vi "M04 Smart Grid.vi"(11 "EV3 in":T1) -> (3 "EV3 out":T1)   [LabVIEW 2016]
uses:
  <vilib>/NXT/Subs/LVHSConnector.ctl
  <vilib>/NXT/LegoClasses/BrickReference/BrickReference.lvclass
  <vilib>/NXT/Block Support/NXT_OutputPort.ctl
  <vilib>/NXT/NXTIO Xnodes/NXTIONodeSubVIs/NXTMotorRunDistance.vi
  <vilib>/NXT/NXTIO Xnodes/AddressXNode/NXTIOAddress.xnode
  <vilib>/NXT/NXTIO Xnodes/NXTIOXNode/NXTIO.xnode
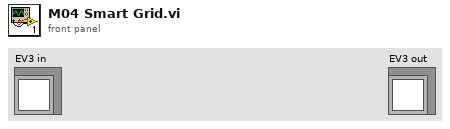
[diagram p1: front panel]
types:
  T1 = typedef "LVHSConnector.ctl" = refnum<class "BrickReference.lvclass">
  T2 = typedef "NXT_OutputPort.ctl" = u8
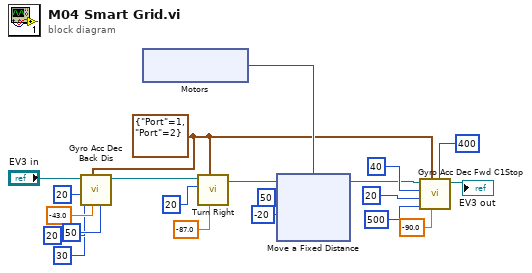
[diagram p0: block diagram]
diagram:
  w6 = cluster{"Port":T2, "Port":T2} {"Port"=1, "Port"=2} ("Motor")
  n1 = call "Gyro Acc Dec Back Dis.vi"("Stop rotation"=50, "Ini. Degrees"=sgl -43.0, "Motor"=w6, "Threshold to De-acc"=20, "De-acc"=20, "Acc"=30, "EV3 in"="EV3 in") -> ("EV3 out"=w8:T1)  [unwired: 4 in]
  n2 = xnode "Motors"() -> ("Motor"=w17:T2)
  n3 = call "Turn Right.vi"("Turning angle"=sgl -87.0, "Motor"=w6, "Motor B (right)"=i8 20, "EV3 in"=w8) -> ("EV3 out"=w18:T1)  [unwired: 7 in]
  n4 = xnode "Move a Fixed Distance"("Speed 1"=i8 -20, "Distance 1"=50, "Motors"=w17, "NXT/EV3"=w18) -> ("NXT/EV3"=w11:T1)
  n5 = call "Gyro Acc Dec Fwd C1Stop.vi"("Threshold to C1"=400, "Ini. Degrees"=sgl -90.0, "Motor"=w6, "Threshold to De-acc"=500, "De-acc"=20, "Acc"=40, "EV3 in"=w11) -> ("EV3 out"=→"EV3 out":T1)  [unwired: 3 in, 1 out]
